vi "HNE Page Manager (Next).vi"(3 "error in (no error)":errorcluster) -> (0 "error out":errorcluster, 1 "Next Page":string)   [LabVIEW 2013]
doc: "Reads the Page Manager and returns the name of the next page to be displayed by the HNE"
uses:
  _SubVIs/TypeDefs/Page Operation.ctl
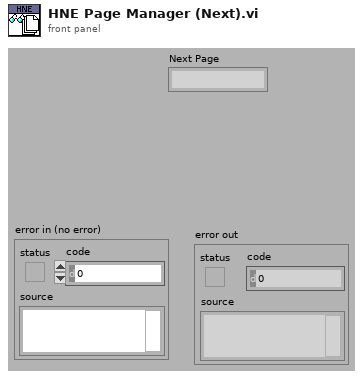
[diagram p1: front panel]
types:
  T1 = typedef "Page Operation.ctl" = enum16{"Init", "Set Next", "Get Next", "Back"}
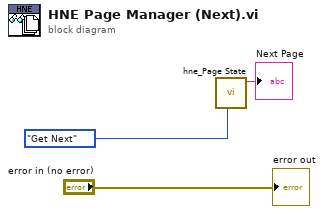
[diagram p0: block diagram]
diagram:
  n1 = call "hne_Page State.vi"("Page Operation"=Page_Operation."Get Next") -> ("Next Page"=→"Next Page":string)  [unwired: 3 in, 7 out]
  "error out" <- "error in (no error)"
